vi "P116ZeroWriteAuto.vi"(8 "error in (no error)":errorcluster) -> (0 "error out":errorcluster, 1 "RateSP(C/min) 2":T2, 2 "NuevoSP(C) 2":T2, 9 "RateSP(C/min)":T2, 10 "NuevoSP(C)":T2)   [LabVIEW 2013]
uses:
  4xP116.ctl
  Controles/P2018 Com Control.ctl
  Eurotherm_Hardware_Module Control.ctl
  P2022 TB INCAR GLOBALES.vi
panel:
  in  "Comunicaciones":T1={"Flujo_1"="ASRL6::INSTR", "Brk1"=FALSE, "Flujo_2"="ASRL6::INSTR", "Brk2"=FALSE, "Flujo_3"="ASRL6::INSTR", "Brk3"=FALSE, "Flujo_4"="ASRL6::INSTR", "Brk4"=FALSE, "Eurothe"="ASRL6::INSTR", "Eurot"=FALSE, "Balanza"="ASRL6::INSTR", "Bal"=FALSE, "eValPos"="ASRL6::INSTR", "eVal"=FALSE, "flowbus"="ASRL6::INSTR", "fb"=FALSE}
  out "TempPV(C)":T2
  out "WorkingSP(C)":T2
  out "TargetSP(C)":T2
  in  "Cancel":bool
  in  "Write":bool
  out "Enable(T)":bool=TRUE
  out "VISA Eurotherm":refnum<visa-resource-name>
  in  "Delay Time (s)":dbl=0.1
  # "Programando controladores P116"
  # "Precal"
  # "Lecho"
  # "Cinta"
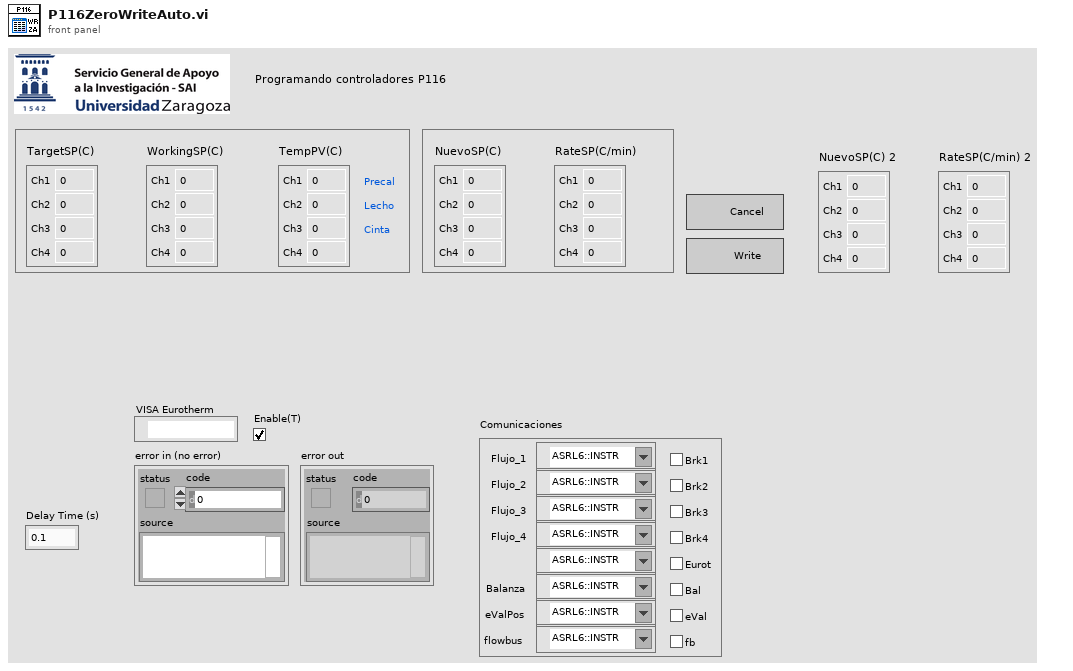
[diagram p1: front panel]
types:
  T1 = typedef "P2018 Com Control.ctl" = cluster{"Flujo_1":refnum<visa-resource-name>, "Brk1":bool, "Flujo_2":refnum<visa-resource-name>, "Brk2":bool, "Flujo_3":refnum<visa-resource-name>, "Brk3":bool, "Flujo_4":refnum<visa-resource-name>, "Brk4":bool, "Eurothe":refnum<visa-resource-name>, "Eurot":bool, "Balanza":refnum<visa-resource-name>, "Bal":bool, "eValPos":refnum<visa-resource-name>, "eVal":bool, "flowbus":refnum<visa-resource-name>, "fb":bool}
  T2 = typedef "4xP116.ctl" = cluster{"Ch1":dbl, "Ch2":dbl, "Ch3":dbl, "Ch4":dbl}
  T3 = typedef "P2018 Eurotherm Control.ctl" = cluster{"TargetSP":T2, "WorkingSP":T2, "Temperatura":T2, "Error":bool, "Date":string, "Delay(s)":dbl, "RateSP":T2, "Potencia":T2}
  T4 = typedef "Eurotherm_Hardware_Module Control.ctl" = enum16{"Initialize", "Write SP", "Read SP+PV", "Write Rate", "Set P", "Set I", "Set D", "Shutdown"}
  T5 = enum16{"Add 1", "Add 2", "Add 10", "Add 11", "Add 12", "Add 13"}[]
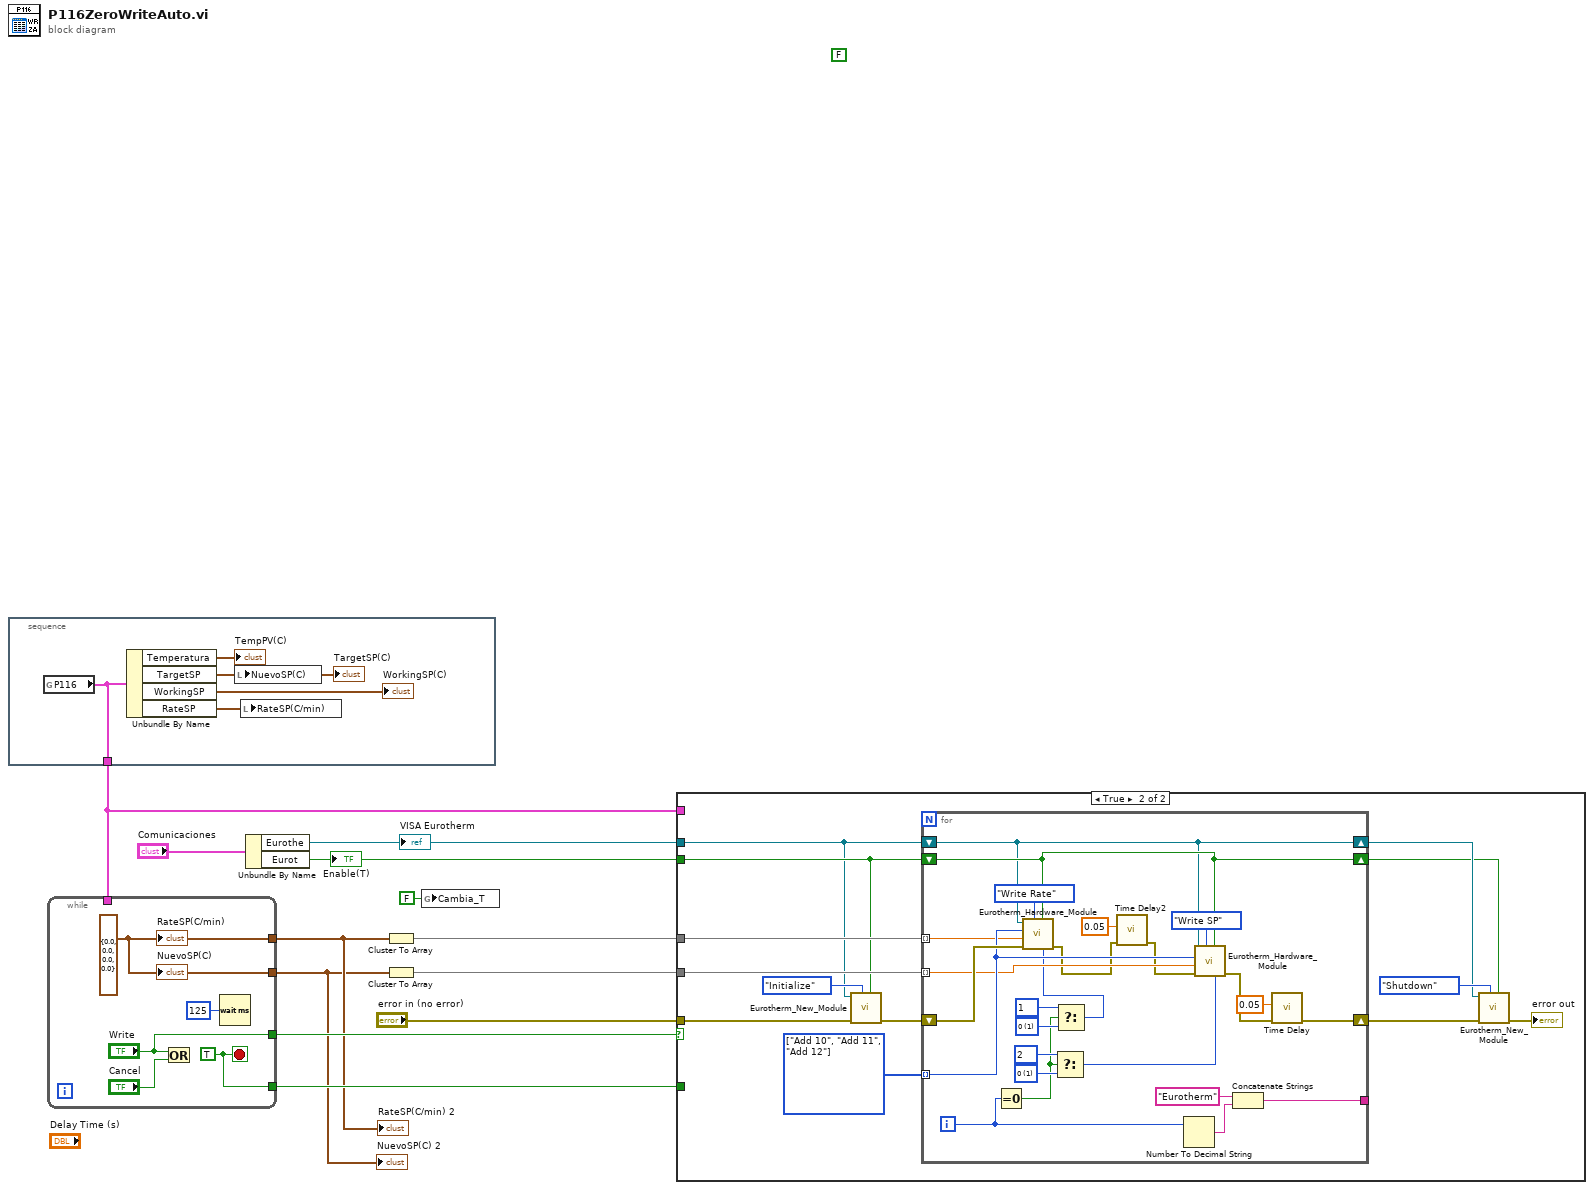
[diagram p0: block diagram]
diagram:
  (unwired) FALSE
  n1 = stacked-sequence {
    tunnel: [w14] -> w4
    frame #0 {
      n2 = global read "P2022 TB INCAR GLOBALES.vi" "P116"() -> (w14:T3)
      n3 = Unbundle By Name(w14) -> ("Temperatura"=→"TempPV(C)":T2, "TargetSP"=w15:T2, "WorkingSP"=→"WorkingSP(C)":T2, "RateSP"=w13:T2)
      "TargetSP(C)" <- w15
      n4 = local write "NuevoSP(C)"(w15) -> ()
      n5 = local write "RateSP(C/min)"(w13) -> ()
    }
  }
  n6 = while {
    tunnel: [w18] -> w11
    tunnel: [w20] -> w2
    tunnel: [w20] -> w3
    tunnel: ["Write"] -> w7
    tunnel: w4 -> [_]
    stop <- w18 stop-if-true
    w20 = T2 {"Ch1"=0.0, "Ch2"=0.0, "Ch3"=0.0, "Ch4"=0.0} ("RateSP(C/min)")
    w18 = TRUE
    n7 = Or(x="Write", y="Cancel") -> ()  [unwired: 1 out]
    n8 = Wait (ms)(milliseconds to wait=u32 125) -> ()  [unwired: 1 out]
    "RateSP(C/min)" <- w20
    "NuevoSP(C)" <- w20
  }
  "NuevoSP(C) 2" <- w2
  "RateSP(C/min) 2" <- w3
  n9 = Unbundle By Name("Comunicaciones") -> ("Eurothe"=w5:refnum<visa-resource-name>, "Eurot"=w12:bool)
  "Enable(T)" <- w12
  "VISA Eurotherm" <- w5
  n10 = Cluster To Array(cluster=w3) -> (array=w8:dbl[])
  n11 = Cluster To Array(cluster=w2) -> (array=w9:dbl[])
  n12 = global write "P2022 TB INCAR GLOBALES.vi" "Cambia_T"(FALSE ("ChangeT")) -> ()
  n13 = case shown="True" w7 {
    tunnel: w12 -> [_ w29]
    tunnel: w11 -> [_ _]
    tunnel: "error in (no error)" -> [_ w31]
    tunnel: w9 -> [_ w34]
    tunnel: w8 -> [_ w35]
    tunnel: w5 -> [_ w28]
    tunnel: w4 -> [_ _]
    frame False {
    }
    frame True {
      w33 = T5 [enum."Add 10", enum."Add 11", enum."Add 12"] items=["Add 1", "Add 2", "Add 10", "Add 11", "Add 12", "Add 13"]
      n14 = call "Eurotherm_New_Module.vi"("Eurotherm (T:Enable)"=w29, "Command"=Eurotherm_Hardware_Module_Control."Initialize", "error in (no error)"=w31, "VISA resource name"=w28) -> ("error out"=w30:errorcluster)  [unwired: 6 in, 1 out]
      n15 = for {
        tunnel: w33 -> [w54] mode=indexing
        shift-right: [w49] -> w24
        shift-left: w30 -> [w55]
        tunnel: [w58] -> _
        tunnel: w34 -> [w51] mode=indexing
        tunnel: w35 -> [w52] mode=indexing
        shift-right: [w39] -> w26
        shift-left: w28 -> [w39]
        shift-right: [w40] -> w25
        shift-left: w29 -> [w40]
        i -> [w45]
        w44 = u16 1 items=["0"=1, "1"=10, "2"=100] ("Decimales")
        w43 = u16 10 items=["0"=1, "1"=10, "2"=100] ("Decimales")
        w47 = u16 1 items=["0"=1, "1"=10, "2"=100] ("Decimales")
        w48 = u16 100 items=["0"=1, "1"=10, "2"=100] ("Decimales")
        n16 = Equal To 0?(x=w45) -> (x = 0?=w41:bool)
        n17 = Select(t=w48, s=w41, f=w47) -> (s? t:f=w46:u16)
        n18 = Select(t=w43, s=w41, f=w44) -> (s? t:f=w42:u16)
        n19 = call "Eurotherm_Hardware_Module.vi"("Decimales"=w42, "Eurotherm (T:Enable)"=w40, "Command"=Eurotherm_Hardware_Module_Control."Write Rate", "error in (no error)"=w55, "Value"=w52, "Address"=w54, "VISA resource name"=w39) -> ("error out"=w37:errorcluster)  [unwired: 2 in, 2 out]
        n20 = call "Time Delay2"("error in (no error)"=w37, "Delay Time (s)"=0.05) -> ("error out"=w36:errorcluster)  [unwired: 9 in]
        n21 = Number To Decimal String(number=w45) -> (decimal integer string=w59:string)  [unwired: 1 in]
        n22 = call "Eurotherm_Hardware_Module.vi"("Decimales"=w46, "Eurotherm (T:Enable)"=w40, "Command"=Eurotherm_Hardware_Module_Control."Write SP", "error in (no error)"=w36, "Value"=w51, "Address"=w54, "VISA resource name"=w39) -> ("error out"=w50:errorcluster)  [unwired: 2 in, 2 out]
        n23 = Concatenate Strings("Eurotherm" ("error source (\" \")"), w59) -> (w58:string)
        n24 = call "Time Delay"("error in (no error)"=w50, "Delay Time (s)"=0.05) -> ("error out"=w49:errorcluster)  [unwired: 9 in]
      }
      n25 = call "Eurotherm_New_Module.vi"("Eurotherm (T:Enable)"=w25, "Command"=Eurotherm_Hardware_Module_Control."Shutdown", "error in (no error)"=w24, "VISA resource name"=w26) -> ("error out"=→"error out":errorcluster)  [unwired: 6 in, 1 out]
    }
  }
